vi "Check Flowmeter.vi"(0 "MW100":refnum<visa-resource-name>="MW100", 2 "Semiphore":T1, 5 "Read? (Write=F)":bool=TRUE, 7 "Turbine Flow?":bool, 11 "Error In":errorcluster) -> (4 "Turbine Flowmeter Settings":bool, 6 "Mag Flowmeter Settings":bool, 14 "Gain, Offset, Threshold":dbl[](array[numeric]), 15 "Error Out":errorcluster)   [LabVIEW 2009]
uses:
  ChannelSettings.ctl
panel:
  out "Half In Mag Settings":bool
  # "A001 020.GT.A003\t%Watt totalizer debouncer math\nA002 TLOG.SUM(A001)\t%Watt totalizer debouncer math\nA003 020*K01\t\t%Watt totalizer debouncer math\n\nA004 018.GT.K05   \t%K05 IS THE THRESHOLD VALUE. 018 IS THE SENSOR INPUT CHANNEL.\nA005 A004*K02*(018-K03) %K03 AND K02 ARE LINEAR SCALING\nA006 A005*C001        \t%C001 IS THE ENABLE FOR TOTALIZING\nA007 TLOG.SUM(A006)\t%INEGRATION\nA008 A007/K04\t\t%SCALE FOR SAMPLING\nA009 A011+A012+A013+A014+A015+A016+A017+A018+A019+A020\nA010 A009/K06\t\t%MOVING AVERAGE OF FLOW\nA011 A012\nA012 A013\nA013 A014\nA015 A016\nA016 A017\nA017 A018\nA018 A019\nA019 A020\nA020 A005"
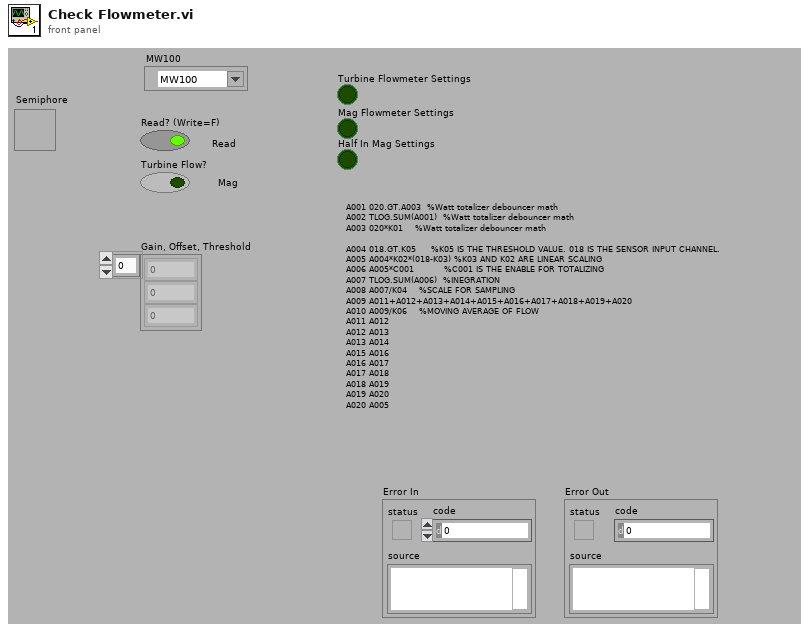
[diagram p1: front panel]
types:
  T1 = typedef "Semaphore RefNum" = refnum<k1>
  T2 = typedef "ChannelSettings.ctl" = u32
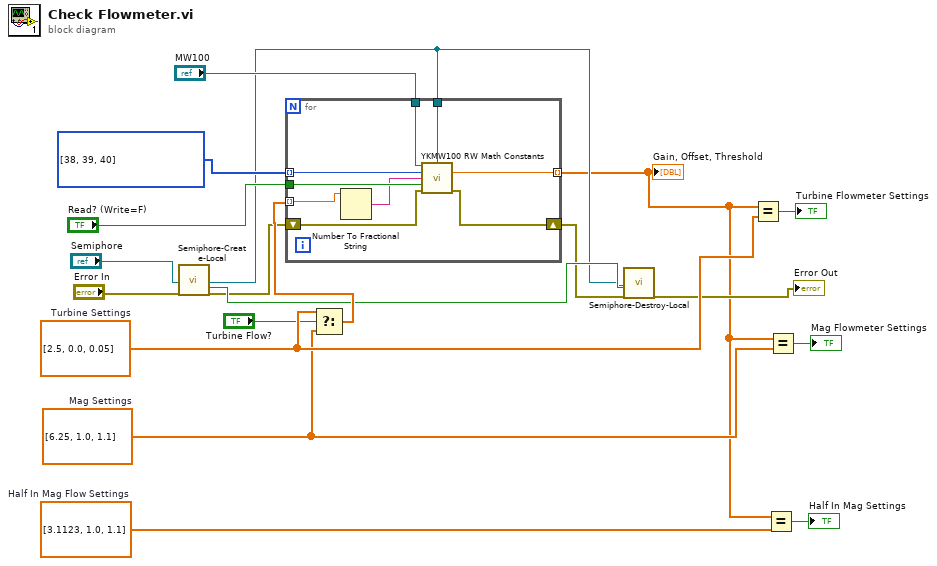
[diagram p0: block diagram]
diagram:
  w2 = dbl[] [3.1123, 1.0, 1.1]  # Half In Mag Flow Settings
  w13 = dbl[] [6.25, 1.0, 1.1]  # Mag Settings
  w14 = dbl[] [2.5, 0.0, 0.05]  # Turbine Settings
  w19 = T2[] [38, 39, 40] items=["4-20_OUT", "Pres_HI1", "Pres_HI2", "Pres_LOW", "Pres_PIN", "HEATER_TOP", "HEATER_BOT", "T_Shell", "FLOWMETER", "WATT_SENSE", "WH_TICK", "Tc_1", "Tc_2", "Tc_3", "Tc_4", "Tc_5", "Tc_6", "Tc_down", "T_Shell_2", "T_Shell_3", "T_Shell_4", "RTD_IN", "RTD_OUT", "RTD_AMB", "INTF_TEMPFLO", "INTF_READY", "INTF_START", "INTF_STOP", "DRM_LOW", "DRM_HIGH", "PWR_MAIN", "VLV_DUMP", "VLV_OUT", "VLV_IN", "WATT_HOURS", "FLOW(SAMPLE)", "GALLONS", "FLOW(GPM)", "FLOW_CALC_GAIN", "FLOW_CALC_OFFSET", "FLOW_CALC_THRESHOLD"]
  n1 = call "Semiphore-Create-Local.vi"("Semiphore"="Semiphore", "error in (no error)"="Error In") -> ("semaphore"=w4:T1, "Local?"=w9:bool, "error out"=w6:errorcluster)  [unwired: 15 in]
  n2 = Select(t=w14, s="Turbine Flow?", f=w13) -> (s? t:f=w11:dbl[])
  n3 = for {
    tunnel: w19 -> [w28] mode=indexing
    tunnel: "MW100" -> [w27]
    tunnel: w4 -> [w26]
    tunnel: [w25] -> w1 mode=indexing
    shift-right: [w23] -> w5
    shift-left: w6 -> [w24]
    tunnel: "Read? (Write=F)" -> [w22]
    tunnel: w11 -> [w21] mode=indexing
    n4 = Number To Fractional String(number=w21) -> (F-format string=w20:string)  [unwired: 3 in]
    n5 = call "YKMW100 RW Math Constants.vi"("MW100"=w27, "Semiphore"=w26, "Channel_Enum"=w28, "Write Value"=w20, "Read? (Write=F)"=w22, "Error In"=w24) -> ("Read Value"=w25:dbl, "Error Out"=w23:errorcluster)  [unwired: 7 in, 1 out]
  }
  "Gain, Offset, Threshold" <- w1
  n6 = call "Semiphore-Destroy-Local.vi"("Semiphore"=w4, "Local?"=w9, "error in (no error)"=w5) -> ("error out"=→"Error Out":errorcluster)  [unwired: 16 in]
  n7 = Equal?(x=w1, y=w14) -> (x = y?=→"Turbine Flowmeter Settings":bool)
  n8 = Equal?(x=w1, y=w2) -> (x = y?=→"Half In Mag Settings":bool)
  n9 = Equal?(x=w1, y=w13) -> (x = y?=→"Mag Flowmeter Settings":bool)
